vi "Run_8_of_8_Tests.vi"() -> ()   [LabVIEW 2019]
uses:
  <vilib>/Rock Robotics/WPI/ThirdParty/JAS_Junk/TrajLib/Trajectory_Library.lvlib
panel:
  out "April Tag":bool
  out "Elevator Sim":bool
  out "Elliptical Region\nConstraint":bool
  out "Trapezoid Profile":bool
  out "String":string
  out "All Tests Finished":bool
  # "FORMAL TRAJECTORY / CONTROL LIBRARY TEST PROCEDURE"
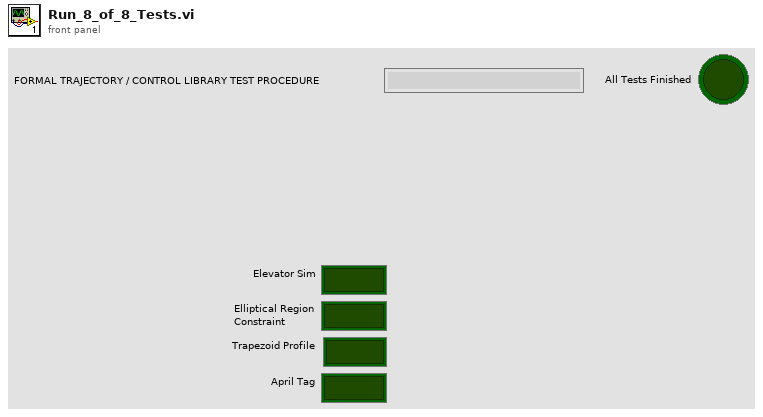
[diagram p1: front panel]
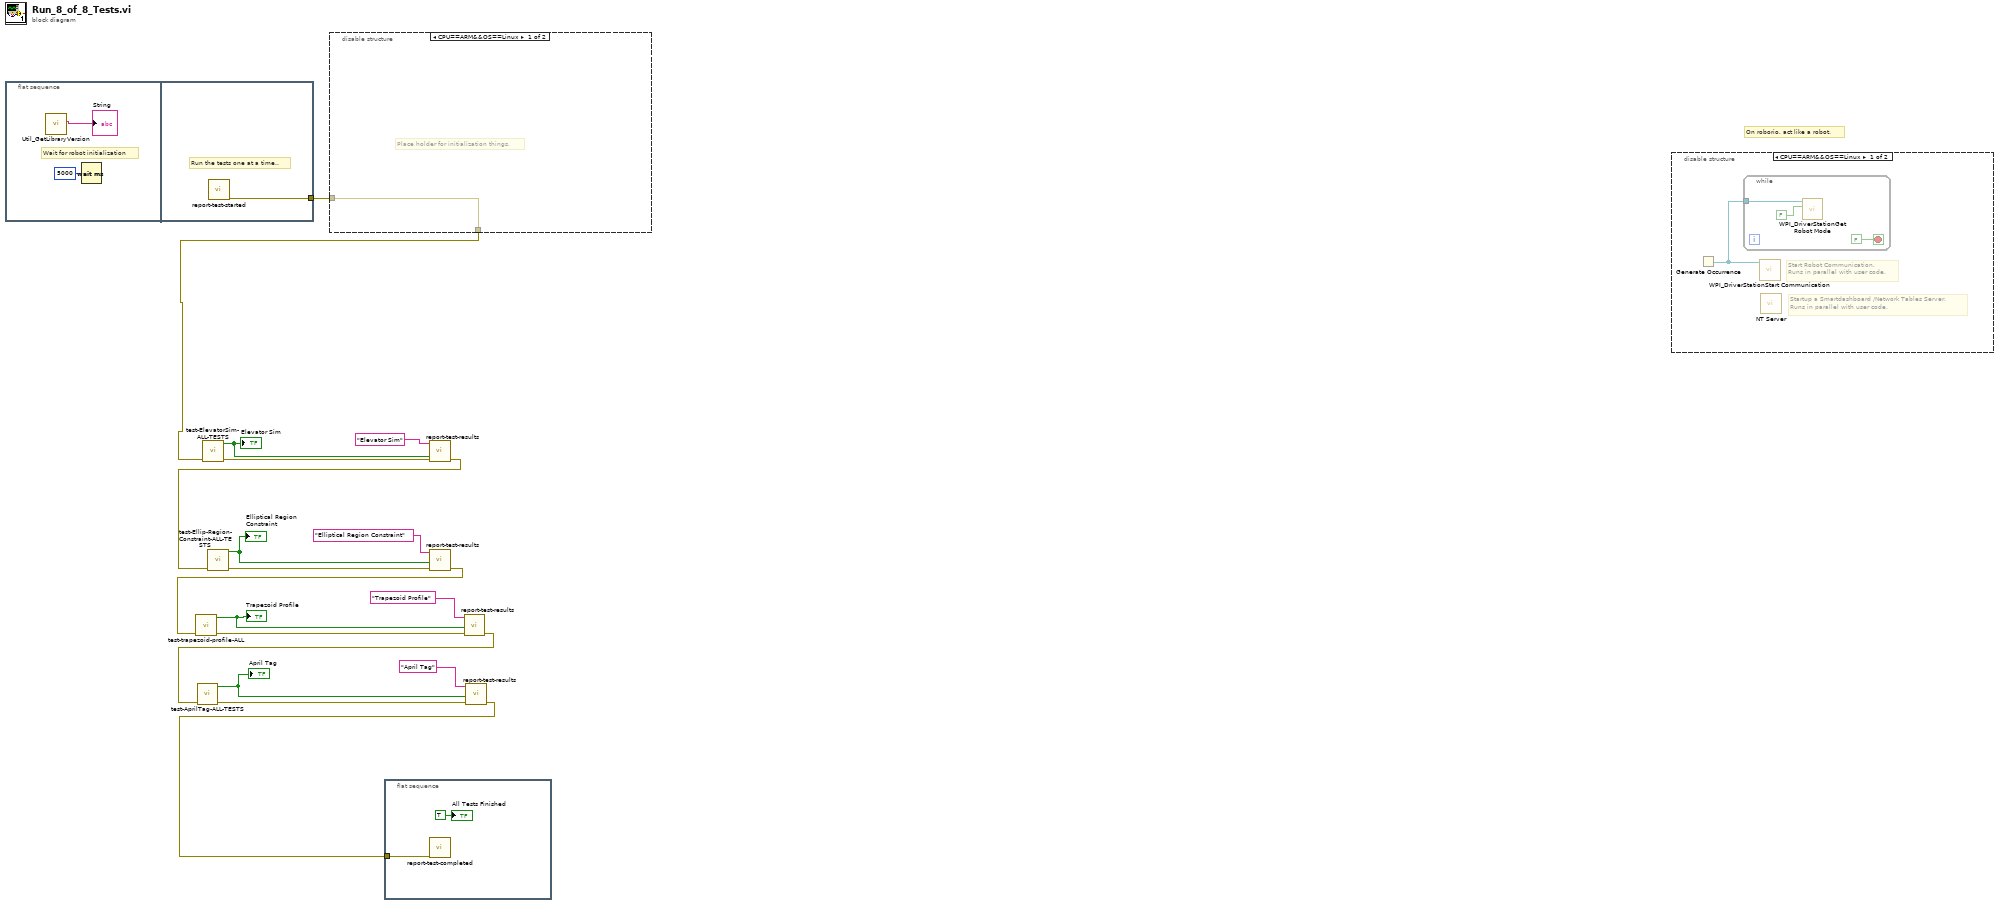
[diagram p0: block diagram]
diagram:
  # "On roborio, act like a robot."
  n1 = flat-sequence {
    tunnel: [w21] -> w18
    frame #0 {
      # "Wait for robot initialization"
      n2 = call <vilib>:"Util_GetLibraryVersion.vi"() -> ("TrajLibVersion"=→"String":string)  [unwired: 11 in]
      n3 = Wait (ms)(milliseconds to wait=u32 5000) -> ()  [unwired: 1 out]
    }
    frame #1 {
      # "Run the tests one at a time.."
      n4 = call "report-test-started.vi"() -> ("error out"=w21:errorcluster)  [unwired: 11 in]
    }
  }
  n5 = disable-structure shown="CPU==ARM&&OS==Linux" {
    disable-tunnel: w18 -> [w22 w23]
    disable-tunnel: [w22 w23] -> w6
    frame condition #0 {
      # "Place holder for initialization things."
    }
    frame condition #1 (active) {
    }
  }
  n6 = call "test-ElevatorSim-ALL-TESTS.vi"("error in (no error)"=w6) -> ("error out"=w8:errorcluster, "All Passed"=w9:bool)  [unwired: 9 in]
  "Elevator Sim" <- w9
  n7 = flat-sequence {
    tunnel: w2 -> [w24]
    frame #0 {
      n8 = call "report-test-completed.vi"("error in (no error)"=w24) -> ()  [unwired: 10 in, 1 out]
      "All Tests Finished" <- TRUE ("All Tests Finished")
    }
  }
  n9 = call "report-test-results.vi"("error in (no error)"=w8, "TestPassed"=w9, "Test Name"="Elevator Sim") -> ("error out"=w7:errorcluster)  [unwired: 8 in]
  n10 = call "test-Ellip-Region-Constraint-ALL-TESTS.vi"("error in (no error)"=w7) -> ("error out"=w13:errorcluster, "All Passed"=w12:bool)  [unwired: 9 in]
  "Elliptical Region\nConstraint" <- w12
  n11 = call "report-test-results.vi"("error in (no error)"=w13, "TestPassed"=w12, "Test Name"="Elliptical Region Constraint") -> ("error out"=w11:errorcluster)  [unwired: 8 in]
  n12 = call "test-trapezoid-profile-ALL.vi"("error in (no error)"=w11) -> ("error out"=w15:errorcluster, "All TEsts passed"=w16:bool)  [unwired: 9 in]
  "Trapezoid Profile" <- w16
  n13 = call "report-test-results.vi"("error in (no error)"=w15, "TestPassed"=w16, "Test Name"="Trapezoid Profile") -> ("error out"=w3:errorcluster)  [unwired: 8 in]
  n14 = call "test-AprilTag-ALL-TESTS.vi"("error in (no error)"=w3) -> ("error out"=w4:errorcluster, "All Passed"=w1:bool)  [unwired: 9 in]
  "April Tag" <- w1
  n15 = call "report-test-results.vi"("error in (no error)"=w4, "TestPassed"=w1, "Test Name"="April Tag") -> ("error out"=w2:errorcluster)  [unwired: 8 in]
  n16 = disable-structure shown="CPU==ARM&&OS==Linux" {
    frame condition #0 {
      # "Startup a Smartdashboard /Network Tables Server.\nRuns in parallel with user code."
      # "Start Robot Communication.\nRuns in parallel with user code."
      n17 = Generate Occurrence() -> (w26:refnum<k4>)
      n18 = while {
        tunnel: w26 -> [w29]
        stop <- FALSE stop-if-true
        n19 = call <vilib>:"WPI_DriverStationGet Robot Mode.vi"("Finish"=FALSE, "DS Occurrence"=w29) -> ()  [unwired: 10 out]
      }
      n20 = call <vilib>:"WPI_DriverStationStart Communication.vi"("occurrence"=w26) -> ()  [unwired: 2 in, 9 out]
      n21 = call <vilib>:"NT Server.vi"() -> ()  [unwired: 12 in]
    }
    frame condition #1 (active) {
    }
  }
